vi "EOL LIN_Send_Single_Message.vi"(0 "NAD":u8=126 format="%.0x", 1 "NeedREQ":bool=TRUE, 2 "CD701 position":bool, 5 "Tx Msg":u8[][](array[numeric]), 7 "LIN Device":T1={"Master Frame(3C)"="MasterReq\nSPA3414_ConfigurationsCMAGeely_CEMCALYPSOSDB34XX0Cfg_LIN3_190709_", "Slave Frame(3D)"="SlaveResp\nSPA3414_ConfigurationsCMAGeely_CEMCALYPSOSDB34XX0Cfg_LIN3_190709_", "Request Schedule"="CEMLIN3DiagRequestSchedule\nSPA3414_ConfigurationsCMAGeely_CEMCALYPSOSDB34XX0Cfg_LIN3_190709_", "Response Schedule"="CEMLIN3DiagResponseSchedule\nSPA3414_ConfigurationsCMAGeely_CEMCALYPSOSDB34XX0Cfg_LIN3_190709_", "Frame Write SCU"="", "Frame Read SCU"="", "LIN Name"=""}, 9 "FrameCount":i32=1, 11 "error in (no error)":errorcluster, 12 "Msg Wait Time":u32=3000, 13 "Retries":i32=5) -> (3 "TxRx Data":string[][](array[string]), 4 "Response Good?":bool, 6 "spreadsheet string":string, 8 "Rx Msg":u8[](array[numeric]) format="%.0x", 15 "error out":errorcluster)   [LabVIEW 2018]
uses:
  LIN Device.ctl
panel:
  out "size(s)":i32
  # "3000  OLD"
  # "5  old"
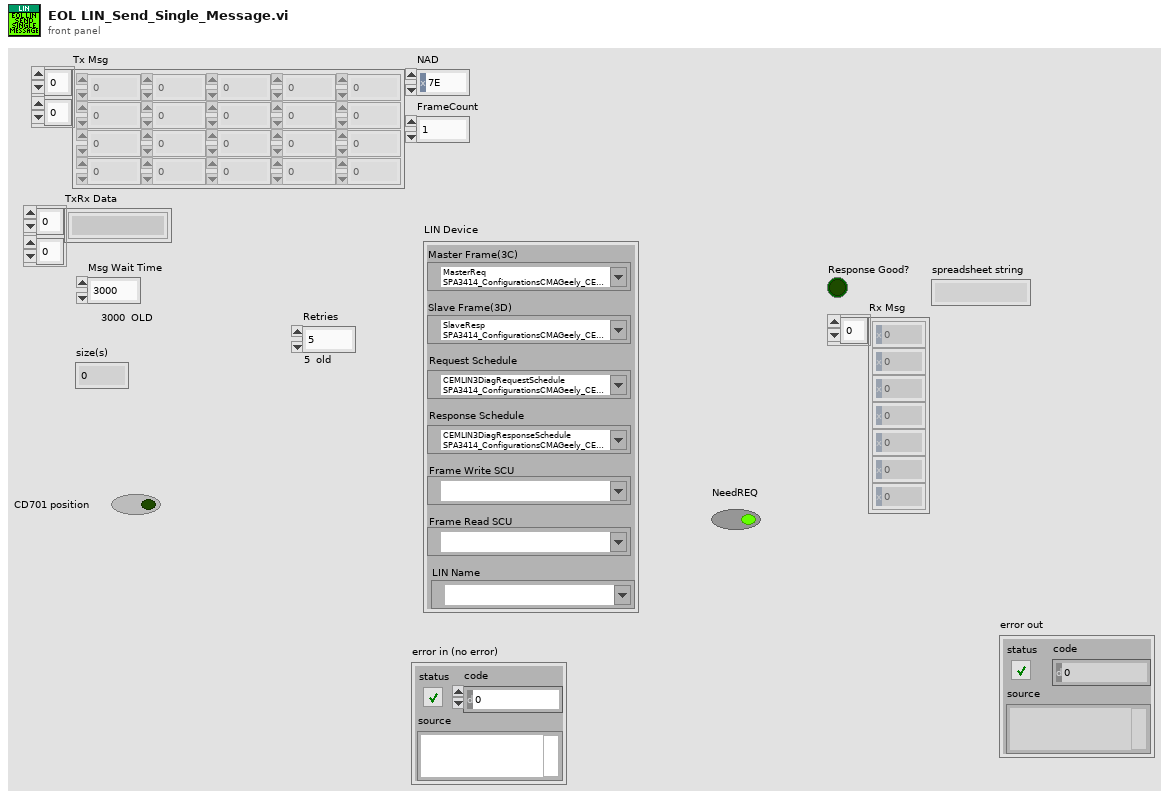
[diagram p1: front panel]
types:
  T1 = typedef "LIN Device.ctl" = cluster{"Master Frame(3C)":refnum<k21>, "Slave Frame(3D)":refnum<k21>, "Request Schedule":refnum<k21>, "Response Schedule":refnum<k21>, "Frame Write SCU":refnum<k21>, "Frame Read SCU":refnum<k21>, "LIN Name":refnum<k21>}
  T2 = cluster{"Tx Msg":u8[][], "NAD":u8, "Retry Counter":i32, "Rx Msg":u8[], "FrameCount":i32, "FF":u8[], "Response Good?":bool, "TxRx Data":string[][], "Message Start Timer":u32, "LIN Device":T1, "element":string[]}
  T3 = typedef "XNET Frame LIN.ctl" = cluster{"timestamp":timestamp, "payload":u8[], "identifier":u32, "type":T4, "event ID":u8, "event slot?":bool, "echo?":bool}
  T4 = typedef "XNET Frame Type LIN.ctl" = u8
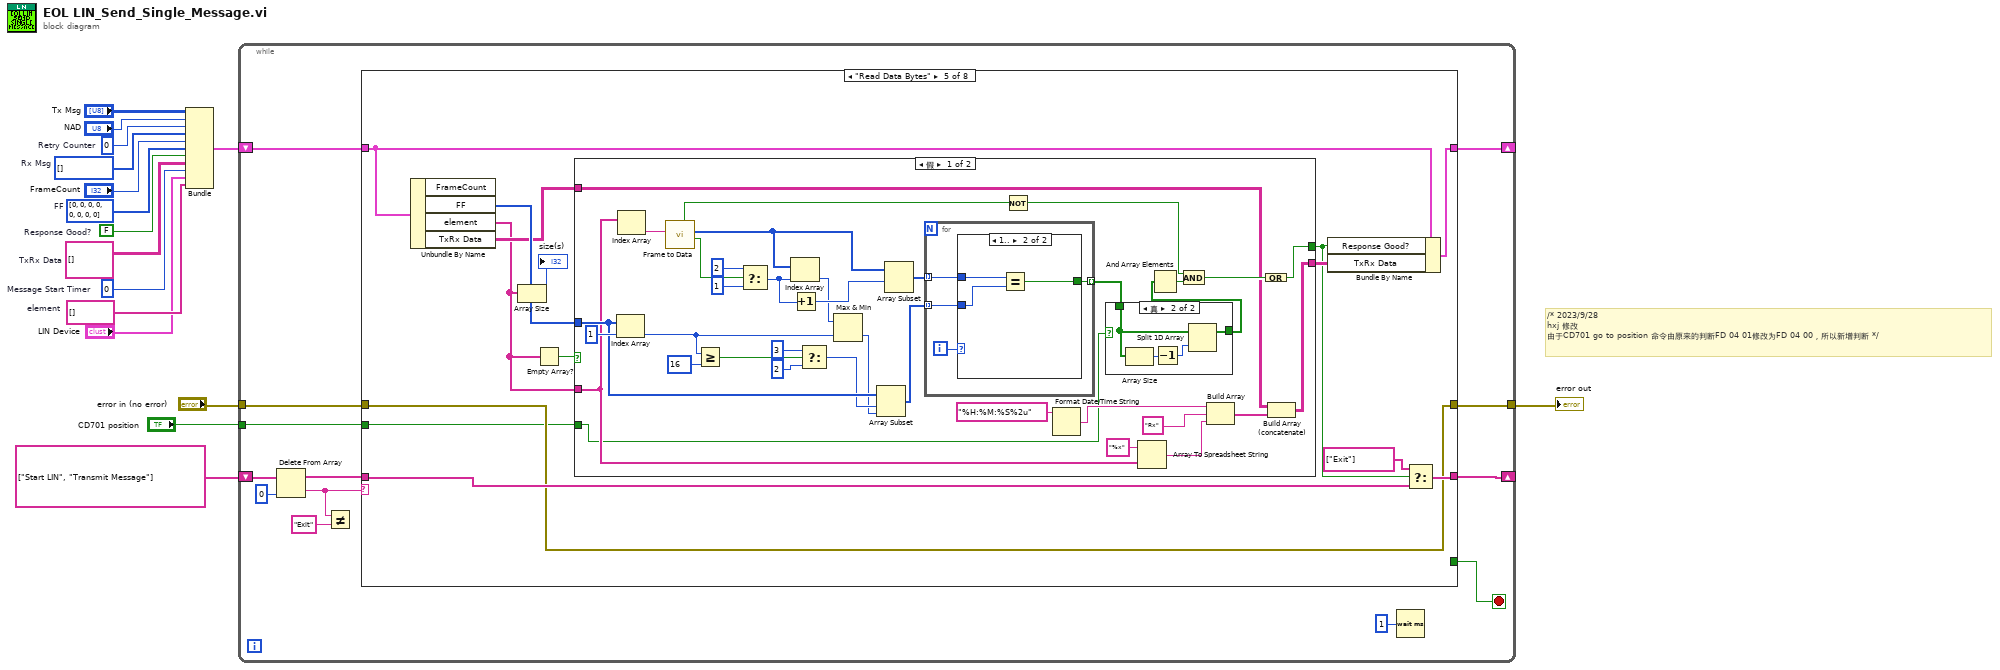
[diagram p0: block diagram]
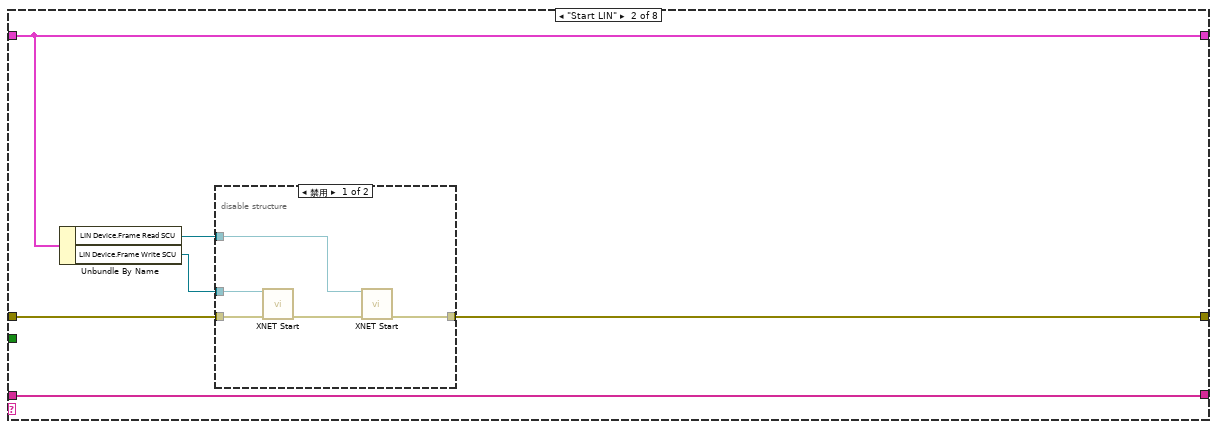
[diagram p3: hidden frame]
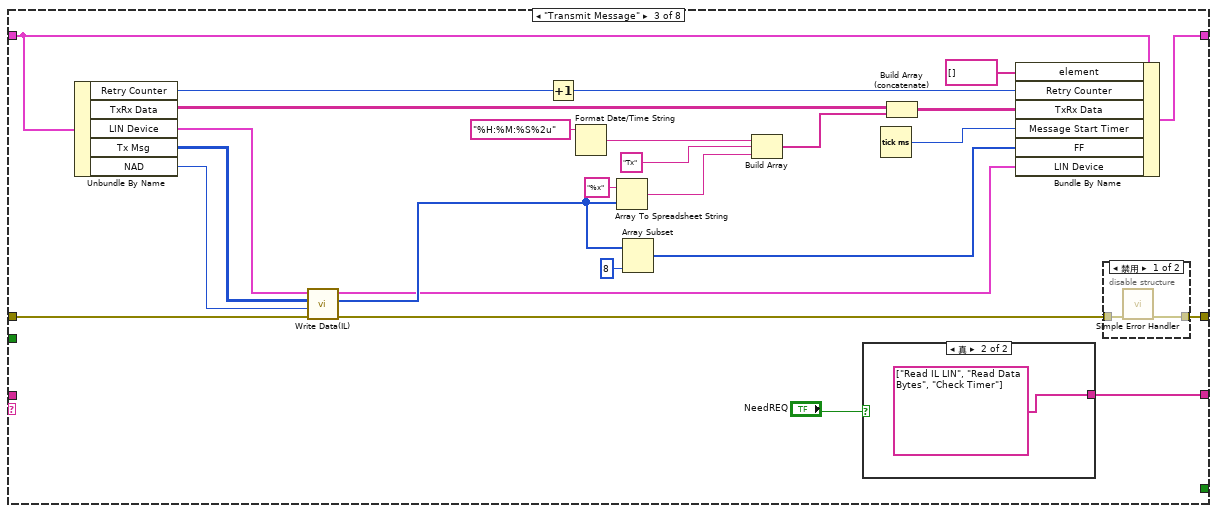
[diagram p5: hidden frame]
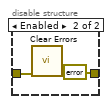
[diagram p6: hidden frame]
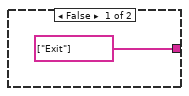
[diagram p7: hidden frame]
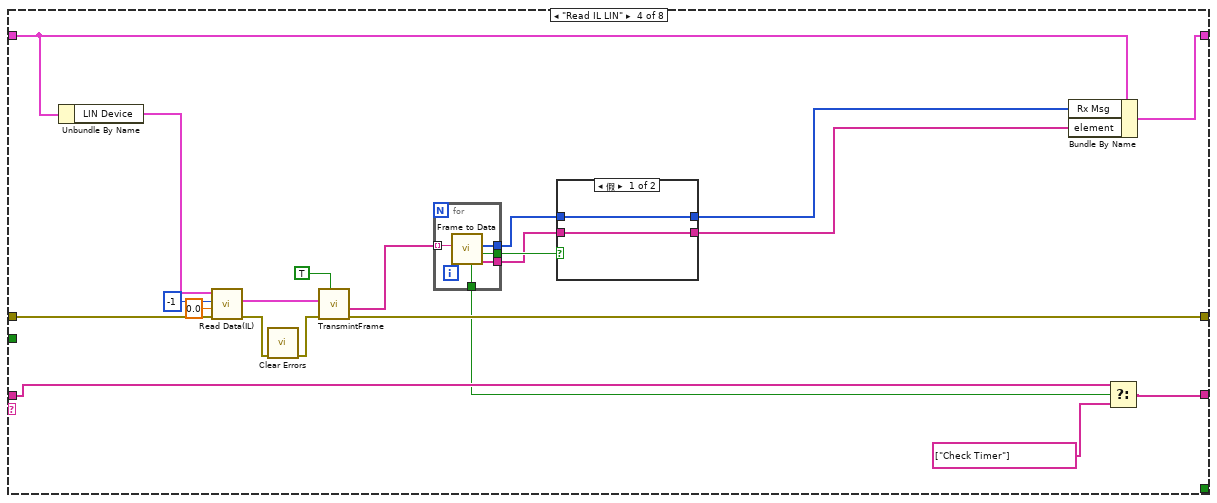
[diagram p8: hidden frame]
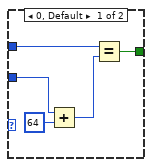
[diagram p11: hidden frame]
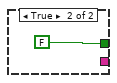
[diagram p12: hidden frame]
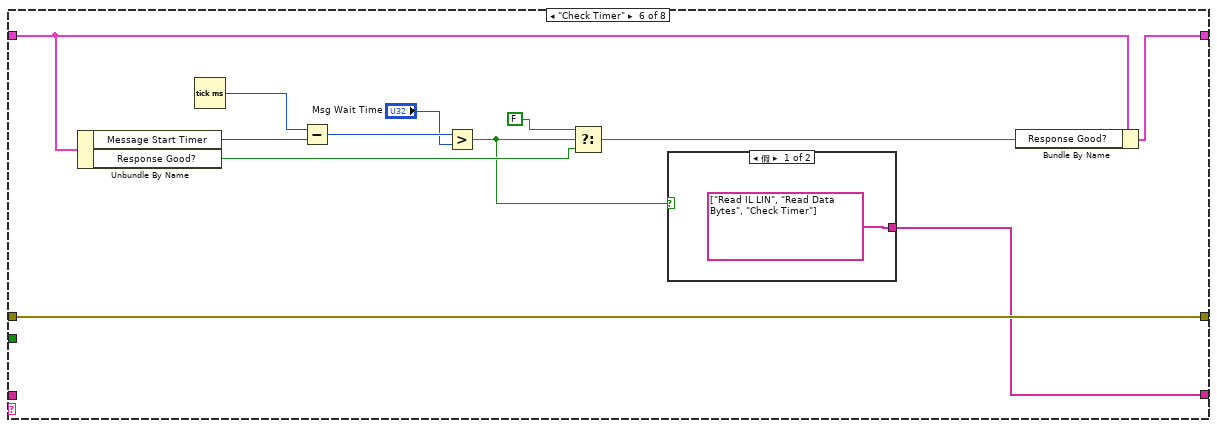
[diagram p13: hidden frame]
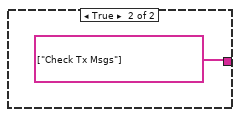
[diagram p14: hidden frame]
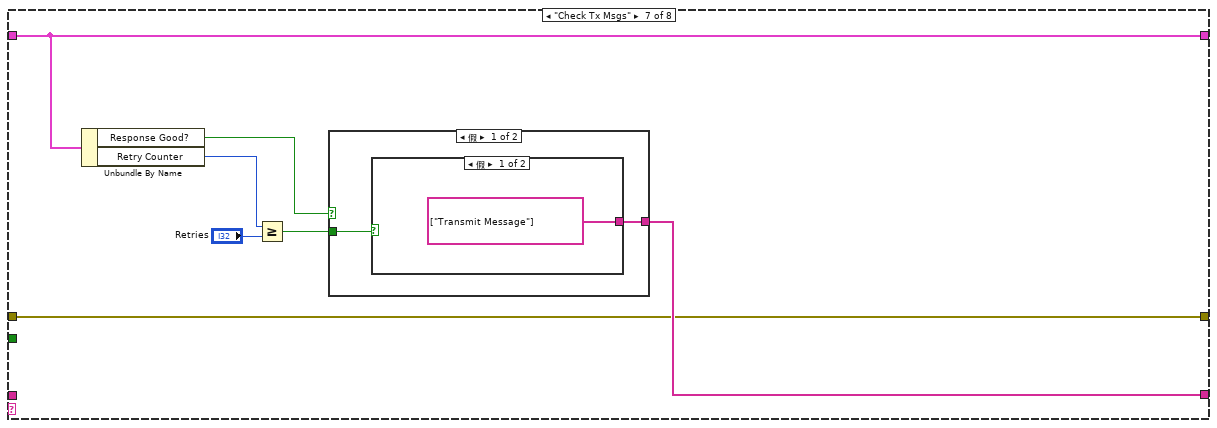
[diagram p15: hidden frame]
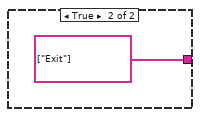
[diagram p16: hidden frame]
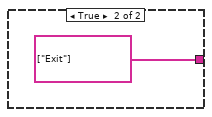
[diagram p17: hidden frame]
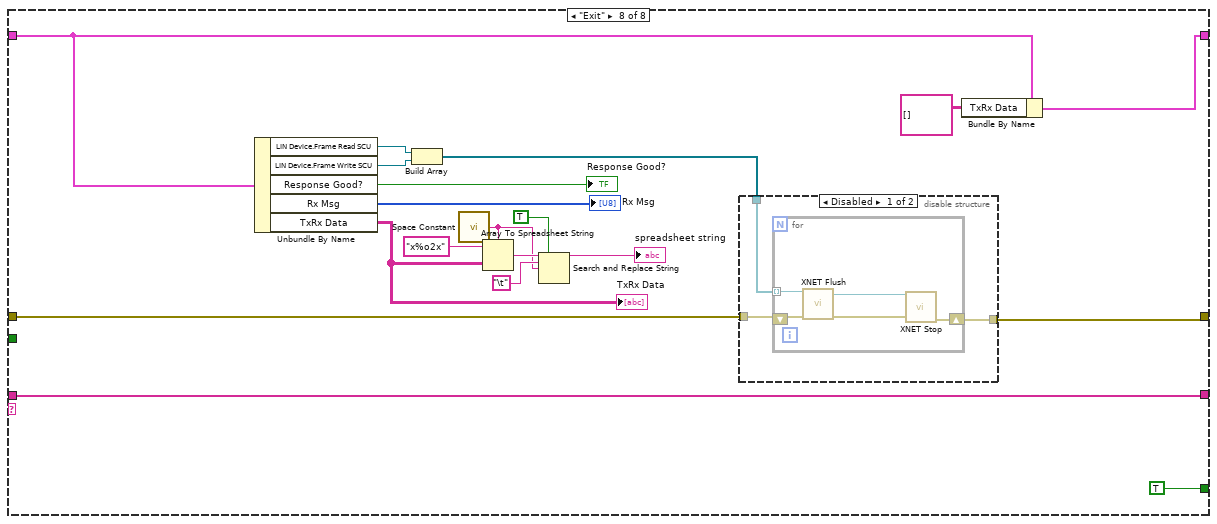
[diagram p18: hidden frame]
diagram:
  w6 = string[] []  # element
  w7 = u32 0  # Message Start Timer
  w9 = FALSE  # Response Good?
  w8 = string[][] []  # TxRx Data
  w10 = u8[] [0, 0, 0, 0, 0, 0, 0, 0]  # FF
  w12 = u8[] []  # Rx Msg
  w13 = 0  # Retry Counter
  # "/* 2023/9/28\nhxj 修改\n由于CD701 go to position 命令由原来的判断FD 04 01修改为FD 04 00，所以新增判断 */"
  n1 = Bundle("Tx Msg"="Tx Msg", "NAD"="NAD", "Retry Counter"=w13, "Rx Msg"=w12, "FrameCount"="FrameCount", "FF"=w10, "Response Good?"=w9, "TxRx Data"=w8, "Message Start Timer"=w7, "LIN Device"="LIN Device", "element"=w6) -> (w5:T2)  [unwired: 1 in]
  n2 = while {
    shift-right: [w29] -> _
    shift-left: w5 -> [w28]
    shift-right: [w27] -> _
    shift-left: string[] ["Start LIN", "Transmit Message"] -> [w22]
    tunnel: "error in (no error)" -> [w26]
    tunnel: [w25] -> w3
    tunnel: "CD701 position" -> [w17]
    stop <- w24 stop-if-true
    n3 = Delete From Array(array=w22, index=0) -> (deleted portion=w20:string, array with subset deleted=w23:string[])  [unwired: 1 in]
    n4 = Not Equal?(x=w20, y="Exit") -> ()  [unwired: 1 out]
    n5 = case shown="\"Read Data Bytes\"" w20 {
      tunnel: w23 -> [w31 w33 _ w88 w113 _ _ w215]
      tunnel: [w32 w35 w45 w92 w119 w186 w191 w218] -> w29
      tunnel: w28 -> [w32 w35 w70 w93 w120 w185 w191 w216]
      tunnel: [w31 w33 w51 w90 w114 w175 w190 w215] -> w27
      tunnel: w26 -> [w30 w38 w69 w97 w110 w184 w189 w208]
      tunnel: [w30 w34 w57 w91 w110 w184 w189 w207] -> w25
      tunnel: [_ _ _ _ _ _ _ TRUE] -> w24
      tunnel: w17 -> [_ _ _ _ w107 _ _ _]
      frame "Error", Default {
      }
      frame "Start LIN" {
        n6 = Unbundle By Name(w35) -> ("LIN Device.Frame Read SCU"=w36:refnum<k21>, "LIN Device.Frame Write SCU"=w37:refnum<k21>)
        n7 = disable-structure shown="禁用" {
          disable-tunnel: w38 -> [w43 w44]
          disable-tunnel: w37 -> [w42 _]
          disable-tunnel: w36 -> [w40 _]
          disable-tunnel: [w39 w44] -> w34
          frame Disabled {
            n8 = call <vilib>:"XNET Start.vi"("session in"=w42, "error in (no error)"=w43) -> ("error out"=w41:errorcluster)  [unwired: 12 in, 1 out]
            n9 = call <vilib>:"XNET Start.vi"("session in"=w40, "error in (no error)"=w41) -> ("error out"=w39:errorcluster)  [unwired: 12 in, 1 out]
          }
          frame Enabled {
          }
        }
      }
      frame "Transmit Message" {
        n10 = Unbundle By Name(w70) -> ("Retry Counter"=w66:i32, "TxRx Data"=w63:string[][], "LIN Device"=w50:T1, "Tx Msg"=w68:u8[][], "NAD"=w67:u8)
        n11 = call "Write Data(IL).vi"("error in (no error)"=w69, "NAD"=w67, "Tx Msg"=w68, "LIN Device in"=w50) -> ("error out"=w48:errorcluster, "Array"=w56:u8[], "LIN Device out"=w49:T1)  [unwired: 5 in]
        n12 = Increment(x=w66) -> (x+1=w64:i32)
        n13 = Format Date/Time String(time format string (%c)="%H:%M:%S%2u") -> (date/time string=w46:string)  [unwired: 2 in]
        n14 = Array To Spreadsheet String(array=w56, 3:"%x") -> (spreadsheet string=w59:string)  [unwired: 1 in]
        n15 = Array Subset(array=w56, length=8) -> (w54:u8[])  [unwired: 1 in]
        n16 = Build Array(w46, "Tx", w59) -> (w58:string[])
        n17 = case shown="真" "NeedREQ" {
          tunnel: [string[] ["Exit"] string[] ["Read IL LIN", "Read Data Bytes", "Check Timer"]] -> w51
          frame False {
          }
          frame True {
          }
        }
        n18 = Tick Count (ms)() -> (millisecond timer value=w53:u32)
        n19 = Build Array (concatenate)(w63, w58) -> (w62:string[][])
        n20 = Bundle By Name(cluster=w70, "element"=string[] [], "Retry Counter"=w64, "TxRx Data"=w62, "Message Start Timer"=w53, "FF"=w54, "LIN Device"=w49) -> (w45:T2)
        n21 = disable-structure shown="禁用" {
          disable-tunnel: [w72 errorcluster {"status"=FALSE, "code"=0, "source"=""} ("error out")] -> w57
          disable-tunnel: w48 -> [w71 w74]
          frame Disabled {
            n22 = call <vilib>:"Simple Error Handler.vi"("error in (no error)"=w71) -> ("error out"=w72:errorcluster)  [unwired: 4 in, 4 out]
          }
          frame Enabled {
            n23 = call <vilib>:"Clear Errors.vi"("error in (no error)"=w74) -> ()  [unwired: 5 in, 2 out]
          }
        }
      }
      frame "Read IL LIN" {
        n24 = Unbundle By Name(w93) -> ("LIN Device"=w96:T1)
        n25 = call "Read Data(IL).vi"("error in (no error)"=w97, "timeout (0)"=0.0, "number to read (-1)"=-1, "LIN Device in"=w96) -> ("error out"=w81:errorcluster, "data"=w95:T3[])  [unwired: 4 in, 2 out]
        n26 = call <vilib>:"Clear Errors.vi"("error in (no error)"=w81) -> ("error out"=w80:errorcluster)  [unwired: 5 in, 1 out]
        n27 = call "TransmintFrame.vi"("Hex and Dec"=TRUE, "error in (no error)"=w80, "data"=w95) -> ("error out"=w91:errorcluster, "DataByte"=w77:string[])  [unwired: 6 in, 1 out]
        n28 = for {
          tunnel: w77 -> [w102] mode=indexing
          tunnel: [w101] -> w87
          tunnel: [w100] -> w86
          tunnel: [w99] -> w85
          tunnel: [w98] -> w84
          n29 = call "Frame to Data.vi"("Frame"=w102) -> ("element"=w98:string[], "MulFrame"=w100:bool, "Array"=w99:u8[], "Finish"=w101:bool)  [unwired: 5 in, 2 out]
        }
        n30 = case shown="假" w86 {
          tunnel: w85 -> [w104 w105]
          tunnel: w84 -> [w103 w106]
          tunnel: [w103 w106] -> w83
          tunnel: [w104 w105] -> w82
          frame False {
          }
          frame True {
          }
        }
        n31 = Bundle By Name(cluster=w93, "Rx Msg"=w82, "element"=w83) -> (w92:T2)
        n32 = Select(t=w88, s=w87, f=string[] ["Check Timer"]) -> (s? t:f=w90:string[])
      }
      frame "Read Data Bytes" {
        n33 = Unbundle By Name(w120) -> ("FF"=w117:u8[], "element"=w109:string[], "TxRx Data"=w116:string[][])  [unwired: 1 out]
        n34 = Array Size(array=w109) -> (size(s)=→"size(s)":i32)
        n35 = Empty Array?(array=w109) -> (empty?=w118:bool)
        n36 = case shown="假" w118 {
          tunnel: w117 -> [w142 _]
          tunnel: w109 -> [w130 _]
          tunnel: [w133 FALSE] -> w112
          tunnel: w116 -> [w127 _]
          tunnel: [w126 _] -> w115
          tunnel: w107 -> [w122 _]
          frame False {
            n37 = Index Array(array=w142, index=1) -> (element=w146:u8)
            n38 = Index Array(array=w130) -> (element=w156:string)  [unwired: 1 in]
            n39 = call "Frame to Data.vi"("Frame"=w156) -> ("MulFrame"=w154:bool, "Array"=w151:u8[], "Error？"=w137:bool)  [unwired: 5 in, 3 out]
            n40 = Greater Or Equal?(x=w146, y=u8 16) -> (x >= y?=w145:bool)
            n41 = Select(t=2, s=w154, f=1) -> (s? t:f=w150:i32)
            n42 = Index Array(array=w151, index=w150) -> (element=w147:u8)
            n43 = Increment(x=w150) -> (x+1=w149:i32)
            n44 = Select(t=3, s=w145, f=2) -> (s? t:f=w141:i32)
            n45 = Max & Min(x=w147, y=w146) -> (min(x,y)=w140:u8)  [unwired: 1 out]
            n46 = Array Subset(array=w142, index=w141, length=w140) -> (w138:u8[])
            n47 = Array Subset(array=w151, index=w149) -> (w139:u8[])  [unwired: 1 in]
            n48 = for {
              tunnel: w139 -> [w164] mode=indexing
              tunnel: w138 -> [w163] mode=indexing
              tunnel: [w162] -> w123 mode=indexing
              i -> [w165]
              n49 = case shown="1.." w165 {
                tunnel: w164 -> [w168 w173]
                tunnel: w163 -> [w170 w172]
                tunnel: [w166 w171] -> w162
                frame 0, Default {
                  n50 = Add(x=w170, y=u8 64) -> (x+y=w167:u8)
                  n51 = Equal?(x=w168, y=w167) -> (x = y?=w166:bool)
                }
                frame 1.. {
                  n52 = Equal?(x=w173, y=w172) -> (x = y?=w171:bool)
                }
              }
            }
            n53 = Not(x=w137) -> (.not. x?=w136:bool)
            n54 = Format Date/Time String(time format string (%c)="%H:%M:%S%2u") -> (date/time string=w124:string)  [unwired: 2 in]
            n55 = case shown="真" w122 {
              tunnel: w123 -> [w157 w159]
              tunnel: [w157 w158] -> w121
              frame False {
              }
              frame True {
                n56 = Array Size(array=w159) -> (size(s)=w160:i32)
                n57 = Decrement(x=w160) -> (x-1=w161:i32)
                n58 = Split 1D Array(array=w159, index=w161) -> (first subarray=w158:bool[])  [unwired: 1 out]
              }
            }
            n59 = Array To Spreadsheet String(array=w130, 3:"%x" ("format string")) -> (spreadsheet string=w129:string)  [unwired: 1 in]
            n60 = And Array Elements(Boolean array=w121) -> (logical AND=w135:bool)
            n61 = Compound Arithmetic op=AND(w136, w135) -> (w134:bool)
            n62 = Build Array(w124, "Rx", w129) -> (w128:string[])
            n63 = Compound Arithmetic op=OR(w134) -> (w133:bool)
            n64 = Build Array (concatenate)(w127, w128) -> (w126:string[][])
          }
          frame True {
          }
        }
        n65 = Bundle By Name(cluster=w120, "Response Good?"=w112, "TxRx Data"=w115) -> (w119:T2)
        n66 = Select(t=string[] ["Exit"], s=w112, f=w113) -> (s? t:f=w114:string[])
      }
      frame "Check Timer" {
        n67 = Unbundle By Name(w185) -> ("Message Start Timer"=w183:u32, "Response Good?"=w177:bool)
        n68 = Tick Count (ms)() -> (millisecond timer value=w182:u32)
        n69 = Subtract(x=w182, y=w183) -> (x-y=w181:u32)
        n70 = Greater?(x=w181, y="Msg Wait Time") -> (0:w176:bool)
        n71 = Select(t=FALSE, s=w176, f=w177) -> (s? t:f=w179:bool)
        n72 = case shown="假" w176 {
          tunnel: [string[] ["Read IL LIN", "Read Data Bytes", "Check Timer"] string[] ["Check Tx Msgs"]] -> w175
          frame False {
          }
          frame True {
          }
        }
        n73 = Bundle By Name(cluster=w185, "Response Good?"=w179) -> (w186:T2)
      }
      frame "Check Tx Msgs" {
        n74 = Unbundle By Name(w191) -> ("Response Good?"=w195:bool, "Retry Counter"=w194:i32)
        n75 = Greater Or Equal?(x=w194, y="Retries") -> (x >= y?=w192:bool)
        n76 = case shown="假" w195 {
          tunnel: w192 -> [w197 _]
          tunnel: [w196 string[] ["Exit"]] -> w190
          frame False {
            n77 = case shown="假" w197 {
              tunnel: [string[] ["Transmit Message"] string[] ["Exit"]] -> w196
              frame False {
              }
              frame True {
              }
            }
          }
          frame True {
          }
        }
      }
      frame "Exit" {
        n78 = Unbundle By Name(w216) -> ("LIN Device.Frame Read SCU"=w210:refnum<k21>, "LIN Device.Frame Write SCU"=w209:refnum<k21>, "Response Good?"=→"Response Good?":bool, "Rx Msg"=→"Rx Msg":u8[], "TxRx Data"=w211:string[][])
        "TxRx Data" <- w211
        n79 = Build Array(w210, w209) -> (w206:refnum<k21>[])
        n80 = call <vilib>:"Space Constant.vi"() -> ("String"=w203:string)
        n81 = Array To Spreadsheet String(delimiter (Tab)=w203, array=w211, 3:"x%o2x") -> (spreadsheet string=w205:string)
        n82 = Search and Replace String(replace all?=TRUE ("替换全部？(F)"), input string=w205, search string="\t", replace string=w203) -> (result string=→"spreadsheet string":string)  [unwired: 4 in, 3 out]
        n83 = disable-structure shown="Disabled" {
          disable-tunnel: w208 -> [w222 w228]
          disable-tunnel: [w221 w228] -> w207
          disable-tunnel: w206 -> [w220 _]
          frame Disabled {
            n84 = for {
              tunnel: w220 -> [w223] mode=indexing
              shift-right: [w224] -> w221
              shift-left: w222 -> [w227]
              n85 = call <vilib>:"XNET Flush.vi"("session in"=w223, "error in (no error)"=w227) -> ("session out"=w225:refnum<k21>, "error out"=w226:errorcluster)  [unwired: 12 in]
              n86 = call <vilib>:"XNET Stop.vi"("session in"=w225, "error in (no error)"=w226) -> ("error out"=w224:errorcluster)  [unwired: 12 in, 1 out]
            }
          }
          frame Enabled {
          }
        }
        n87 = Bundle By Name(cluster=w216, "TxRx Data"=string[][] []) -> (w218:T2)
      }
    }
    n88 = Wait (ms)(milliseconds to wait=u32 1) -> ()  [unwired: 1 out]
  }
  "error out" <- w3
